vi "Stop Core.vi"(10 "final error code":i32 caption="最终错误代码", 11 "Input Operator in":refnum<class "ControlPanel.lvclass"> caption="操作者输入") -> (3 "Input Operator out":refnum<class "ControlPanel.lvclass"> caption="操作者输出")   [LabVIEW 2014, in "ControlPanel.lvlib" / "ControlPanel.lvclass"]
doc: "(<B>文件名</B>：Actor Framework.lvlib:Actor.lvclass:Stop Core.vi)\n\n定义停止前操作者的动作。使用<B>最终错误代码</B>输入判断操作者是否在出错时关闭。\n\n默认情况下，该方法不执行任何动作。子孙类重写该方法，定义出错时的操作，例如，关闭操作者核心方法初始的进程。"
uses:
  ControlPanel.lvclass
  ControlPanel.lvclass/ControlPanel.ctl
  <vilib>/Utility/xml.llb/Write to XML File.vi
  Wrapper_lib/zsActor/ActorWrapper.lvclass
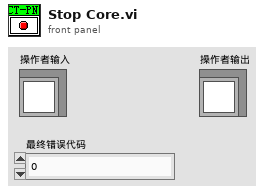
[diagram p1: front panel]
types:
  T1 = typedef "P3AT_Ini.ctl" = cluster{"Is_Dirty":bool, "max_vel":dbl, "max_rot":dbl, "Ini_pose_X":dbl, "Ini_pose_Y":dbl, "Ini_pose_Rot_deg":dbl, "Control_Mode":enum32{"Joy", "Map", "Voice", "Input", "Undefined"}}
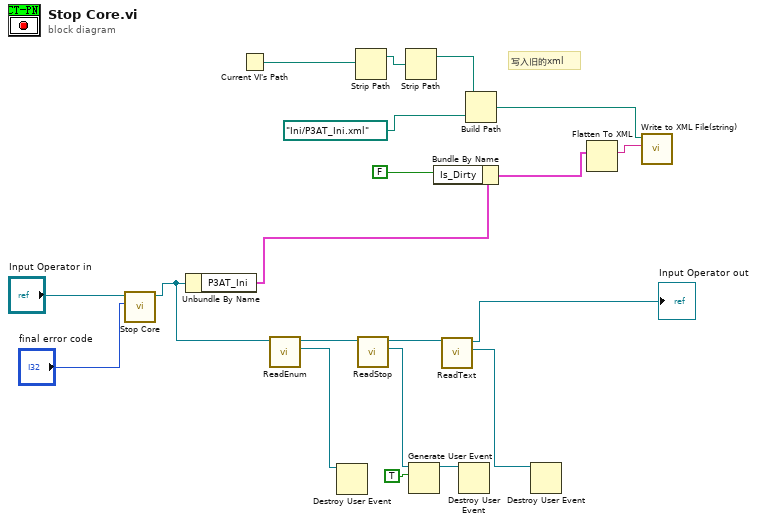
[diagram p0: block diagram]
diagram:
  # "写入旧的xml"
  n1 = call-parent "Stop Core.vi"("final error code"="final error code", "Actor in"="Input Operator in") -> ("Actor out"=w9:refnum<class "ControlPanel.lvclass">)  [unwired: 9 in]
  n2 = Unbundle By Name(w9) -> ("P3AT_Ini"=w10:T1)
  n3 = Current VI's Path() -> (path=w11:path)
  n4 = call-dynamic "ReadEnum.vi"("zsActor输入"=w9) -> ("Enum"=w3:refnum<user-event>, "zsActor输出"=w8:refnum<class "ControlPanel.lvclass">)  [unwired: 8 in, 1 out]
  n5 = Destroy User Event(user event=w3) -> ()  [unwired: 1 in, 1 out]
  n6 = Strip Path(path=w11) -> (stripped path=w17:path)  [unwired: 1 out]
  n7 = call-dynamic "ReadStop.vi"("zsActor输入"=w8) -> ("Stop"=w2:refnum<user-event>, "zsActor输出"=w7:refnum<class "ControlPanel.lvclass">)  [unwired: 8 in, 1 out]
  n8 = Strip Path(path=w17) -> (stripped path=w16:path)  [unwired: 1 out]
  n9 = Generate User Event(user event=w2, event data cluster=TRUE ("event data")) -> (user event out=w4:refnum<user-event>)  [unwired: 2 in, 1 out]
  n10 = Bundle By Name(cluster=w10, "Is_Dirty"=FALSE ("重新定位？")) -> (w12:T1)
  n11 = call-dynamic "ReadText.vi"("zsActor输入"=w7) -> ("Text"=w1:refnum<user-event>, "zsActor输出"=→"Input Operator out":refnum<class "ControlPanel.lvclass">)  [unwired: 8 in, 1 out]
  n12 = Destroy User Event(user event=w4) -> ()  [unwired: 1 in, 1 out]
  n13 = Build Path(base path=w16, name or relative path=path "Ini/P3AT_Ini.xml" ("拆分的路径")) -> (appended path=w14:path)
  n14 = Destroy User Event(user event=w1) -> ()  [unwired: 1 in, 1 out]
  n15 = Flatten To XML(anything=w12) -> (xml string=w18:string)
  n16 = call-poly <vilib>:"Write to XML File(string).vi"("XML Input"=w18, "XML File Path"=w14) -> ()  [unwired: 3 in, 7 out]
